vi "Initialize RGA.vi"(0 "Port Number":refnum<visa-resource-name>, 1 "Timeout Limit":dbl=1.0 format="%.2f", 2 "error in (no error)":errorcluster) -> (3 "Id String":string, 4 "Status Byte":string="\n\r", 5 "Timeout":bool, 6 "error out":errorcluster)   [LabVIEW 2019]
uses:
  Serial Support VISA.llb/Serial Actions.ctl
  Serial Support VISA.llb/Serial port parmeters.ctl
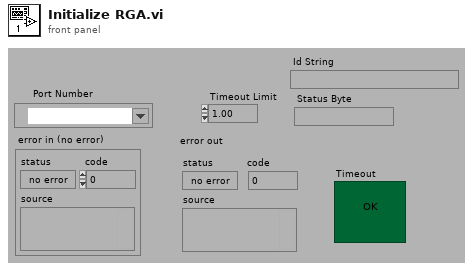
[diagram p1: front panel]
types:
  T1 = typedef "Serial port parmeters.ctl" = cluster{"flow control":enum16{"None", "XON/XOFF", "RTS/CTS"}, "baud rate":u32, "data bits":u16, "Stop Bits":u16, "parity (0:none)":enum16{"None", "Odd", "Even", "Mark", "Space"}, "Transmit Buffer Size":u32, "Receive Buffer Size":u32}
  T2 = typedef "Serial Actions.ctl" = enum16{"Init", "Break", "Clear Buffer", "Write", "Read", "N Bytes", "Lock", "Unlock", "Close"}
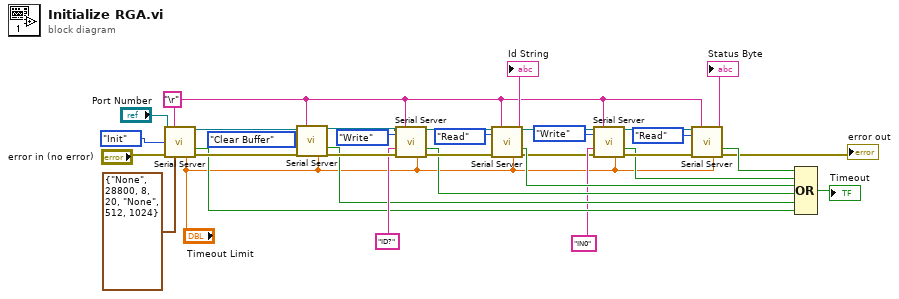
[diagram p0: block diagram]
diagram:
  w15 = "\r" ("EOT Chars (cr/lf)")
  n1 = call "Serial Server.vi"("VISA Resource Name"="Port Number", "EOT Chars (cr/lf)"=w15, "Action"=Serial_Actions."Init", "error in (no error)"="error in (no error)", "Port Parameters"=T1 {"flow control"=enum."None", "baud rate"=28800, "data bits"=8, "Stop Bits"=20, "parity (0:none)"=enum."None", "Transmit Buffer Size"=512, "Receive Buffer Size"=1024}, "Timeout Limit(sec)"="Timeout Limit") -> ("dup VISA Resource Name"=w7:refnum<visa-resource-name>, "Timeout"=w27:bool, "error out"=w32:errorcluster)  [unwired: 5 in, 2 out]
  n2 = call "Serial Server.vi"("VISA Resource Name"=w7, "EOT Chars (cr/lf)"=w15, "Action"=Serial_Actions."Clear Buffer", "error in (no error)"=w32, "Timeout Limit(sec)"="Timeout Limit") -> ("dup VISA Resource Name"=w6:refnum<visa-resource-name>, "Timeout"=w26:bool, "error out"=w31:errorcluster)  [unwired: 6 in, 2 out]
  n3 = call "Serial Server.vi"("VISA Resource Name"=w6, "EOT Chars (cr/lf)"=w15, "Action"=Serial_Actions."Write", "String To Send"="ID?", "error in (no error)"=w31, "Timeout Limit(sec)"="Timeout Limit") -> ("dup VISA Resource Name"=w5:refnum<visa-resource-name>, "Timeout"=w25:bool, "error out"=w28:errorcluster)  [unwired: 5 in, 2 out]
  n4 = call "Serial Server.vi"("VISA Resource Name"=w5, "EOT Chars (cr/lf)"=w15, "Action"=Serial_Actions."Read", "error in (no error)"=w28, "Timeout Limit(sec)"="Timeout Limit") -> ("dup VISA Resource Name"=w4:refnum<visa-resource-name>, "Serial Read"=→"Id String":string, "Timeout"=w24:bool, "error out"=w21:errorcluster)  [unwired: 6 in, 1 out]
  n5 = call "Serial Server.vi"("VISA Resource Name"=w4, "EOT Chars (cr/lf)"=w15, "Action"=Serial_Actions."Write", "String To Send"="IN0", "error in (no error)"=w21, "Timeout Limit(sec)"="Timeout Limit") -> ("dup VISA Resource Name"=w3:refnum<visa-resource-name>, "Timeout"=w18:bool, "error out"=w19:errorcluster)  [unwired: 5 in, 2 out]
  n6 = call "Serial Server.vi"("VISA Resource Name"=w3, "EOT Chars (cr/lf)"=w15, "Action"=Serial_Actions."Read", "error in (no error)"=w19, "Timeout Limit(sec)"="Timeout Limit") -> ("Serial Read"=→"Status Byte":string, "Timeout"=w17:bool, "error out"=→"error out":errorcluster)  [unwired: 6 in, 2 out]
  n7 = Compound Arithmetic op=OR(w17, w18, w24, w25, w26, w27) -> (→"Timeout":bool)
